vi "PXI-Stop AOAI.vi"(0 "AO Tasks":T1[](array[typedef]), 1 "DI Tasks":T1[](array[typedef]), 2 "DO Tasks":T1[](array[typedef]), 5 "AI Tasks":T1[](array[typedef]), 7 "Counter Task":T1, 11 "error in (no error)":errorcluster) -> (15 "error out":errorcluster)   [LabVIEW 2020]
uses:
  Type Defs/Task Struct.ctl
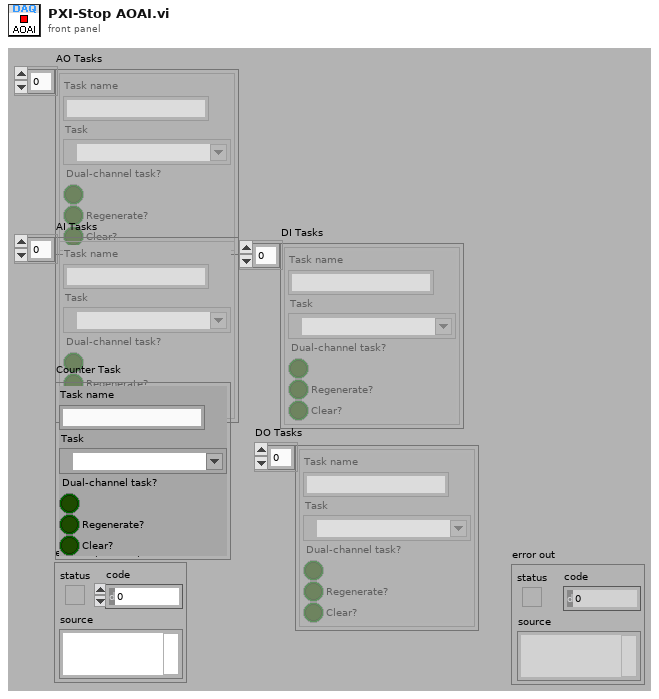
[diagram p1: front panel]
types:
  T1 = typedef "Task Struct.ctl" = cluster{"Task name":string, "Task":refnum<k21>, "Dual-channel task?":bool, "Regenerate?":bool, "Clear?":bool}
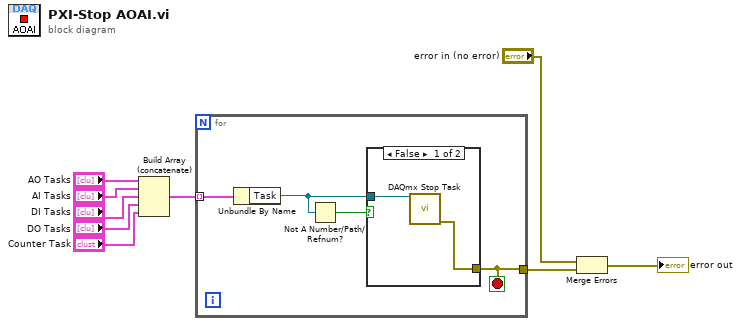
[diagram p0: block diagram]
diagram:
  n1 = Build Array (concatenate)("AO Tasks", "AI Tasks", "DI Tasks", "DO Tasks", "Counter Task") -> (w5:T1[])
  n2 = for {
    tunnel: w5 -> [w13] mode=indexing
    tunnel: [w12] -> w3
    stop <- w12 stop-if-true
    n3 = Unbundle By Name(w13) -> ("Task"=w11:refnum<k21>)
    n4 = Not A Number/Path/Refnum?(number/path/refnum=w11) -> (NaN/Path/Refnum?=w10:bool)
    n5 = case shown="False" w10 {
      tunnel: w11 -> [w15 _]
      tunnel: [w14 _] -> w12
      frame False {
        n6 = call <vilib>:"DAQmx Stop Task.vi"("task/channels in"=w15) -> ("error out"=w14:errorcluster)  [unwired: 13 in, 1 out]
      }
      frame True {
        # "Don't start\nthe Sync task"
      }
    }
  }
  n7 = Merge Errors("error in (no error)", w3) -> (→"error out":errorcluster)
